vi "Load Help File.vi"(8 "error in (no error)":errorcluster, 9 "HTML File":string="MainPage_J1939.html", 10 "Main CHM File":string="J1939.chm", 11 "SHDocVw.IWebBrowser2":refnum<k7>(container)) -> (0 "error out":errorcluster)   [LabVIEW 2018, in "FPGA Addon System Explorer.lvlib"]
uses:
  FPGA Addon System Explorer.lvlib
  <vilib>/Utility/LVLibp/NI_PackedLibraryUtility.lvlib
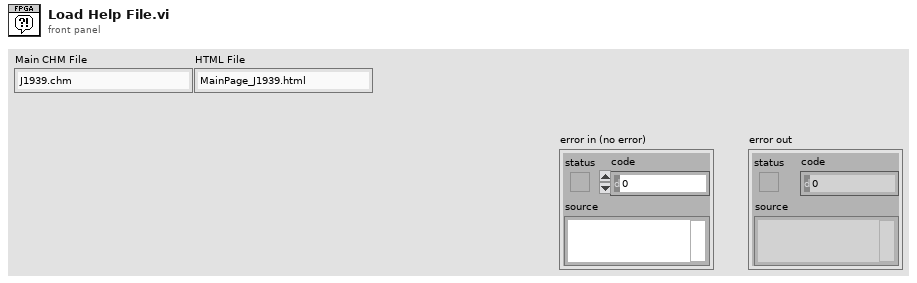
[diagram p1: front panel]
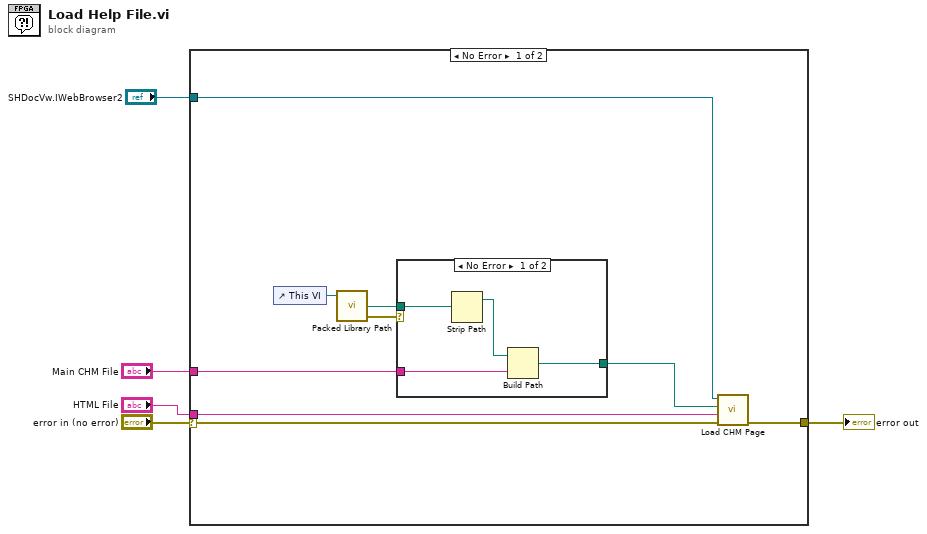
[diagram p0: block diagram]
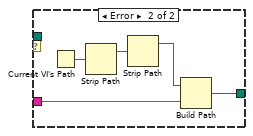
[diagram p2: hidden frame]
diagram:
  n1 = case shown="No Error" "error in (no error)" {
    selector: "error in (no error)" -> [w6 w24]
    tunnel: "HTML File" -> [w14 _]
    tunnel: "Main CHM File" -> [w13 _]
    tunnel: "SHDocVw.IWebBrowser2" -> [w12 _]
    tunnel: [w11 w24] -> w2
    frame No Error {
      n2 = control-ref of="This VI"() -> (w9:refnum<vi>)
      n3 = call <vilib>:"Packed Library Path.vi"("vi reference"=w9) -> ("error out"=w8:errorcluster, "packed library path"=w7:path)  [unwired: 2 in, 1 out]
      n4 = case shown="No Error" w8 {
        tunnel: w13 -> [w17 w20]
        tunnel: [w15 w19] -> w10
        tunnel: w7 -> [w18 _]
        frame No Error {
          n5 = Strip Path(path=w18) -> (stripped path=w16:path)  [unwired: 1 out]
          n6 = Build Path(base path=w16, name or relative path=w17) -> (appended path=w15:path)
        }
        frame Error {
          n7 = Current VI's Path() -> (path=w23:path)
          n8 = Strip Path(path=w23) -> (stripped path=w22:path)  [unwired: 1 out]
          n9 = Strip Path(path=w22) -> (stripped path=w21:path)  [unwired: 1 out]
          n10 = Build Path(base path=w21, name or relative path=w20) -> (appended path=w19:path)
        }
      }
      n11 = call <vilib>:"Load CHM Page.vi"("error in (no error)"=w6, "HTML File"=w14, "Compiled CHM Path"=w10, "Web Browser Reference"=w12) -> ("error out"=w11:errorcluster)  [unwired: 7 in]
    }
    frame Error {
    }
  }
  "error out" <- w2
